vi "RPC__method Template.vi"(8 "error in (no error)":errorcluster, 11 "OOP Server in":refnum<class "OOP Server.lvclass">) -> (0 "error out":errorcluster, 3 "OOP Server out":refnum<class "OOP Server.lvclass">)   [LabVIEW 2019, in "OOP Server.lvclass"]
uses:
  OOP Server.lvclass
  OOP Server.lvclass/OOP Server.ctl
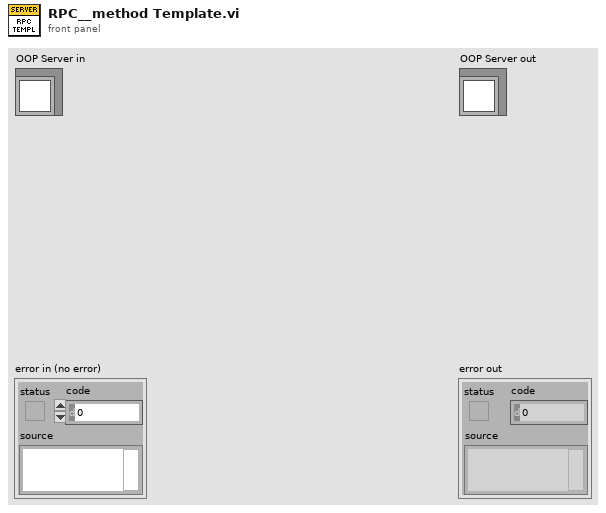
[diagram p1: front panel]
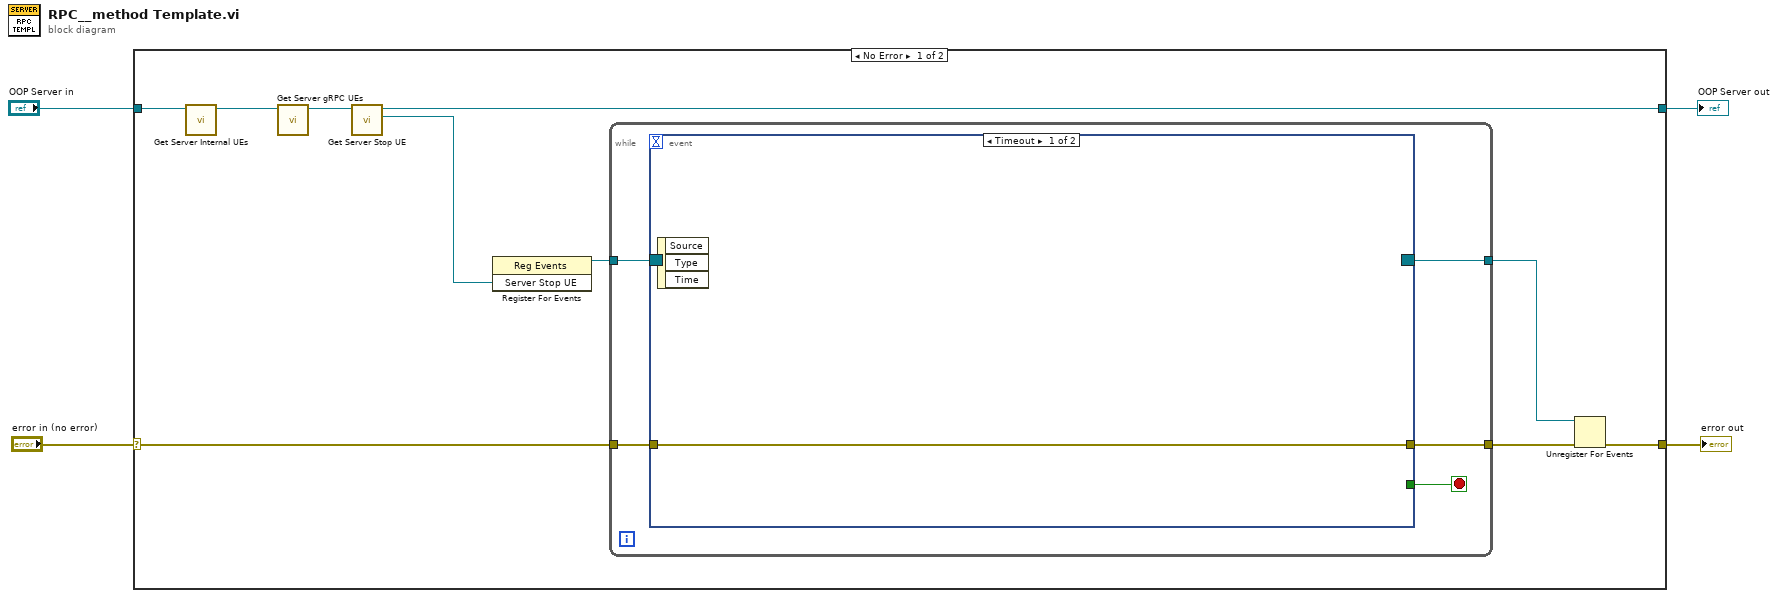
[diagram p0: block diagram]
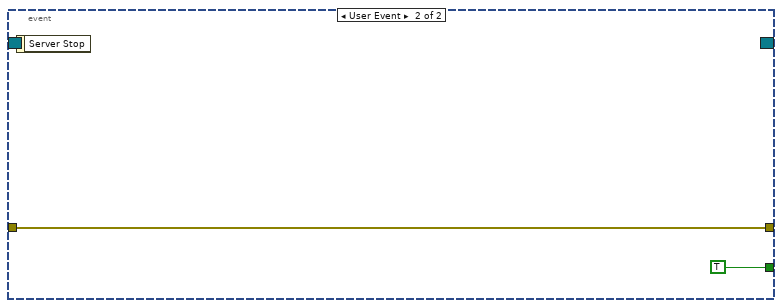
[diagram p2: hidden frame]
diagram:
  n1 = case shown="No Error" "error in (no error)" {
    selector: "error in (no error)" -> [w8 w24]
    tunnel: [w6 w24] -> w3
    tunnel: [w12 w23] -> w1
    tunnel: "OOP Server in" -> [w10 w23]
    frame No Error {
      n2 = call "Get Server Internal UEs.vi"("OOP Server in"=w10) -> ("OOP Server out"=w9:refnum<class "OOP Server.lvclass">)  [unwired: 9 in, 1 out]
      n3 = call "Get Server gRPC UEs.vi"("OOP Server in"=w9) -> ("OOP Server out"=w14:refnum<class "OOP Server.lvclass">)  [unwired: 9 in, 1 out]
      n4 = call "Get Server Stop UE.vi"("OOP Server in"=w14) -> ("Server Stop UE"=w13:refnum<user-event>, "OOP Server out"=w12:refnum<class "OOP Server.lvclass">)  [unwired: 9 in]
      n5 = register-events(w13) -> (reference out=w11:refnum<event-registration>)  [unwired: 2 in, 1 out]
      n6 = while {
        tunnel: w11 -> [w19]
        tunnel: w8 -> [w17]
        tunnel: [w16] -> w7
        tunnel: [w15] -> w5
        stop <- w18 stop-if-true
        n7 = event shown="[0] Timeout" {
          selector: w19 -> [_ _]
          dyn-events: [_ _] -> w15
          timeout: _ -> [_ _]
          tunnel: [_ TRUE] -> w18
          tunnel: w17 -> [w20 w21]
          tunnel: [w20 w21] -> w16
          event Timeout {
            n8 = event-data() -> ()  [unwired: 1 in, 3 out]
          }
          event User Event {
            n9 = event-data() -> ()  [unwired: 1 in, 1 out]
          }
        }
      }
      n10 = Unregister For Events(event registration refnum=w5, error in=w7) -> (error out=w6:errorcluster)
    }
    frame Error {
    }
  }
  "error out" <- w3
  "OOP Server out" <- w1
